vi "Extract ROIs.vi"(8 "error in (no error)":errorcluster, 11 "Retiga in":refnum<class "Retiga.lvclass">) -> (0 "error out":errorcluster, 3 "Retiga out":refnum<class "Retiga.lvclass">)   [LabVIEW 2012, in "Retiga.lvclass"]
uses:
  Retiga.lvclass
  Retiga.lvclass/Retiga.ctl
  <vilib>/vision/NI_Vision_Development_Module.lvlib
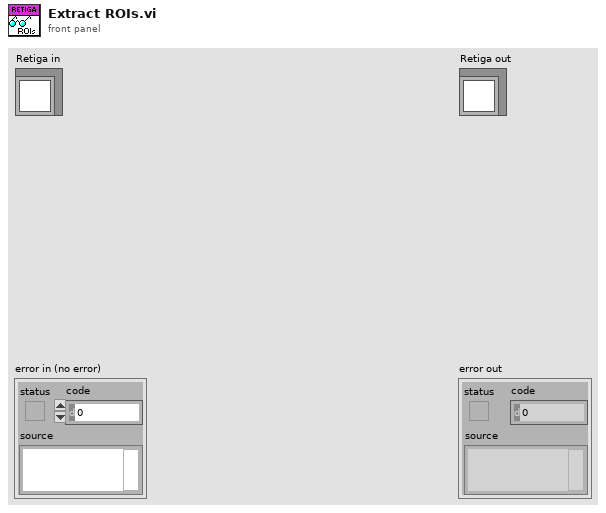
[diagram p1: front panel]
types:
  T1 = typedef "IMAQ Image.ctl" = refnum<image>
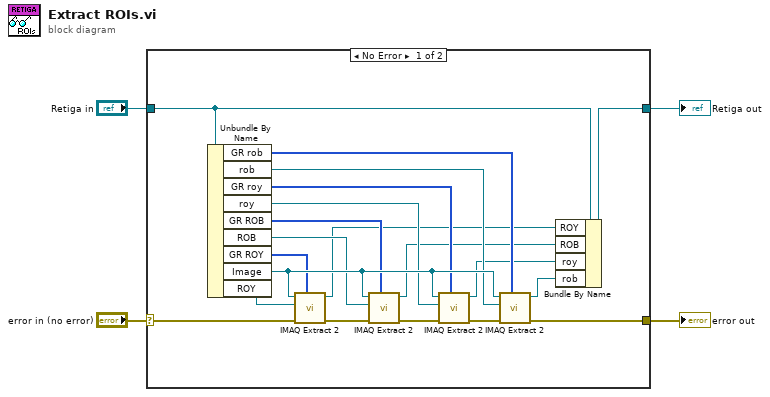
[diagram p0: block diagram]
diagram:
  n1 = case shown="No Error" "error in (no error)" {
    selector: "error in (no error)" -> [w21 w26]
    tunnel: [w20 w26] -> w3
    tunnel: [w9 w25] -> w1
    tunnel: "Retiga in" -> [w10 w25]
    frame No Error {
      n2 = Unbundle By Name(w10) -> ("GR rob"=w14:i32[], "rob"=w11:T1, "GR roy"=w15:i32[], "roy"=w12:T1, "GR ROB"=w16:i32[], "ROB"=w13:T1, "GR ROY"=w17:i32[], "Image"=w18:T1, "ROY"=w19:T1)
      n3 = call "IMAQ Extract 2"("Optional Rectangle"=w17, "error in (no error)"=w21, "Image Dst"=w19, "Image Src"=w18) -> ("error out"=w24:errorcluster, "Image Dst Out"=w8:T1)  [unwired: 6 in]
      n4 = call "IMAQ Extract 2"("Optional Rectangle"=w16, "error in (no error)"=w24, "Image Dst"=w13, "Image Src"=w18) -> ("error out"=w23:errorcluster, "Image Dst Out"=w7:T1)  [unwired: 6 in]
      n5 = call "IMAQ Extract 2"("Optional Rectangle"=w15, "error in (no error)"=w23, "Image Dst"=w12, "Image Src"=w18) -> ("error out"=w22:errorcluster, "Image Dst Out"=w6:T1)  [unwired: 6 in]
      n6 = call "IMAQ Extract 2"("Optional Rectangle"=w14, "error in (no error)"=w22, "Image Dst"=w11, "Image Src"=w18) -> ("error out"=w20:errorcluster, "Image Dst Out"=w5:T1)  [unwired: 6 in]
      n7 = Bundle By Name(cluster=w10, "ROY"=w8, "ROB"=w7, "roy"=w6, "rob"=w5) -> (w9:refnum<class "Retiga.lvclass">)
    }
    frame Error {
    }
  }
  "error out" <- w3
  "Retiga out" <- w1
